vi "Post-Build Custom Action.vi"(10 "Variant":variant) -> (0 "error out":errorcluster)   [LabVIEW 2019]
uses:
  <userlib>/LevyLab/Build Support/PostBuildSupport/PostBuildSupport.lvclass
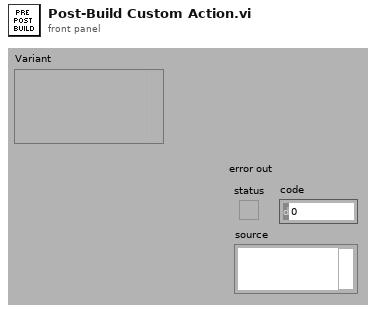
[diagram p1: front panel]
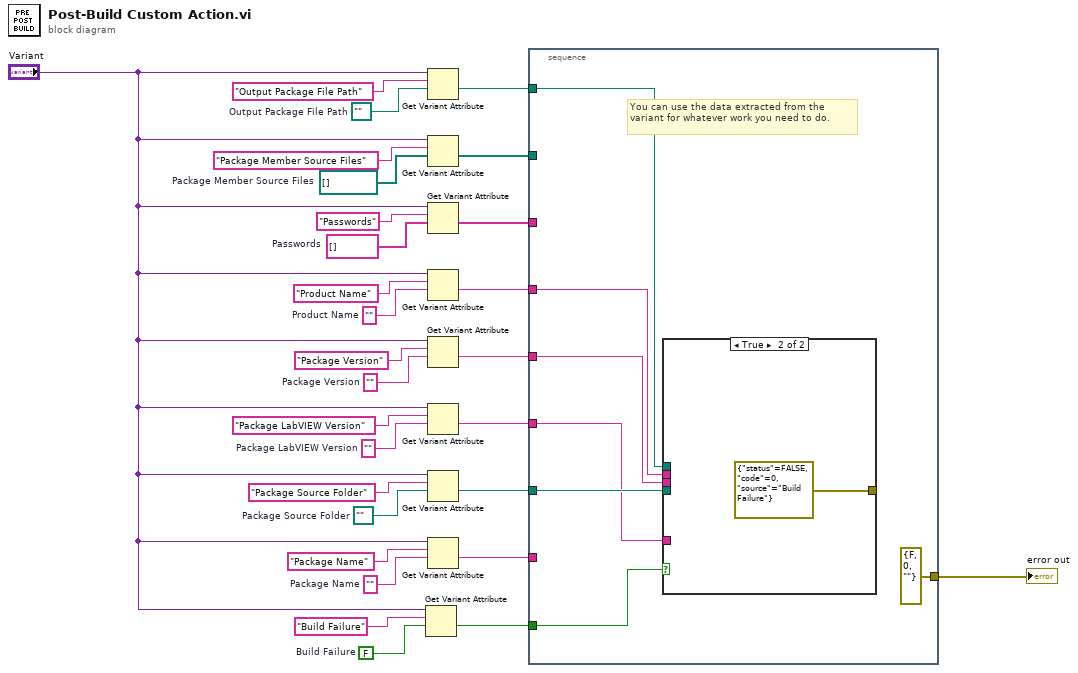
[diagram p0: block diagram]
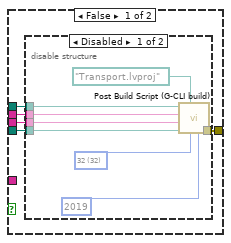
[diagram p2: hidden frame]
diagram:
  w4 = FALSE  # Build Failure
  w14 = path ""  # Package Source Folder
  w15 = ""  # Package Name
  w18 = ""  # Package LabVIEW Version
  w20 = ""  # Package Version
  w22 = ""  # Product Name
  w24 = string[] []  # Passwords
  w26 = path[] []  # Package Member Source Files
  w28 = path ""  # Output Package File Path
  n1 = Get Variant Attribute(Variant="Variant", name="Build Failure", default value (empty Variant)=w4) -> (value=w2:bool)  [unwired: 1 in, 3 out]
  n2 = Get Variant Attribute(Variant="Variant", name="Output Package File Path", default value (empty Variant)=w28) -> (value=w13:path)  [unwired: 1 in, 3 out]
  n3 = Get Variant Attribute(Variant="Variant", name="Package Member Source Files", default value (empty Variant)=w26) -> (value=w12:path[])  [unwired: 1 in, 3 out]
  n4 = Get Variant Attribute(Variant="Variant", name="Passwords", default value (empty Variant)=w24) -> (value=w11:string[])  [unwired: 1 in, 3 out]
  n5 = Get Variant Attribute(Variant="Variant", name="Product Name", default value (empty Variant)=w22) -> (value=w10:string)  [unwired: 1 in, 3 out]
  n6 = Get Variant Attribute(Variant="Variant", name="Package Version", default value (empty Variant)=w20) -> (value=w9:string)  [unwired: 1 in, 3 out]
  n7 = Get Variant Attribute(Variant="Variant", name="Package LabVIEW Version", default value (empty Variant)=w18) -> (value=w8:string)  [unwired: 1 in, 3 out]
  n8 = Get Variant Attribute(Variant="Variant", name="Package Source Folder", default value (empty Variant)=w14) -> (value=w7:path)  [unwired: 1 in, 3 out]
  n9 = Get Variant Attribute(Variant="Variant", name="Package Name", default value (empty Variant)=w15) -> (value=w6:string)  [unwired: 1 in, 3 out]
  n10 = stacked-sequence {
    tunnel: w13 -> [w34]
    tunnel: w12 -> [_]
    tunnel: w11 -> [_]
    tunnel: w10 -> [w33]
    tunnel: w9 -> [w35]
    tunnel: w8 -> [w32]
    tunnel: w7 -> [w36]
    tunnel: w6 -> [_]
    tunnel: w2 -> [w30]
    tunnel: [errorcluster {"status"=FALSE, "code"=0, "source"=""} ("error out")] -> w1
    frame #0 {
      # "You can use the data extracted from the variant for whatever work you need to do."
      n11 = case shown="True" w30 {
        tunnel: w36 -> [w41 _]
        tunnel: w35 -> [w40 _]
        tunnel: w32 -> [_ _]
        tunnel: w34 -> [w39 _]
        tunnel: w33 -> [w38 _]
        tunnel: [w37 errorcluster {"status"=FALSE, "code"=0, "source"="Build Failure"} ("error out")] -> _
        frame False {
          n12 = disable-structure shown="Disabled" {
            disable-tunnel: w41 -> [w49 _]
            disable-tunnel: w40 -> [w48 _]
            disable-tunnel: w39 -> [w46 _]
            disable-tunnel: w38 -> [w45 _]
            disable-tunnel: [w43 _] -> w37
            frame Disabled {
              w47 = u32 32 items=["32"=32, "64"=64] ("Architecture")
              n13 = call <userlib>:"Post Build Script (G-CLI build).vi"(4:u32 2019 ("LV Version"), "Package LabVIEW Version (19.0 (32-bit))"=w47, "Project File Path"=path "Transport.lvproj", "Package Source Folder"=w49, "Package Version (major.minor.patch.build)"=w48, "Product Name"=w45, "Output Package File Path"=w46) -> ("error out"=w43:errorcluster)  [unwired: 4 in]
            }
            frame Enabled {
            }
          }
        }
        frame True {
        }
      }
    }
  }
  "error out" <- w1
